vi "ZLIB Open Zip Archive__ogtk.vi"(4 "error in (no error)":errorcluster, 6 "append (create new)":T1, 7 "archive name":path) -> (0 "error out":errorcluster, 2 "globalComment":string, 3 "zip Refnum":T2)   [LabVIEW 2019]
doc: "Opens a zip session."
uses:
  <userlib>/_OpenG.lib/lvzip/lvzlib.dll
  ZLIB Zip Handle__ogtk.ctl
  ZLIB Open ZIP Mode__ogtk.ctl
panel:
  # "Please visit http://www.OpenG.org to learn about the\nOpen Source LabVIEW software movement.\n\nNOTICE -- YOU MUST LEAVE THIS NOTICE IN PLACE.  PER THE TERMS OF THE LICENSE BELOW, YOU MAY SUBLICENSE THIS SOFTWARE \nIN ANY WAY THAT DOES NOT CONFLICT WITH THIS LICENSE.\n\n### BSD License (http://www.opensource.org/licenses/bsd-license.php) Begin ###\n \nCopyright (C) 2002-2004 Rolf Kalbermatter rolf.kalbermatter@citeng.com\nCopyright (C) 2002 Jim Kring jim@jimkring.com\n\nAll rights reserved.\n\nRedistribution and use in source and binary forms, with or without modification, are permitted provided that the following conditions are met:\n\n    * Redistributions of source code must retain the above copyright notice, this list of conditions and the following disclaimer.\n    * Redistributions in binary form must reproduce the above copyright notice, this list of conditions and the following disclaimer in the \n       documentation and/or other materials provided with the distribution.\n    * Neither the name of SciWare, James Kring, Inc., nor the names of its contributors may be used to endorse or promote products derived \n       from this software without specific prior written permission.\n\nTHIS SOFTWARE IS PROVIDED BY THE COPYRIGHT HOLDERS AND CONTRIBUTORS \"AS IS\" AND ANY EXPRESS OR IMPLIED WARRANTIES, \nINCLUDING, BUT NOT LIMITED TO, THE IMPLIED WARRANTIES OF MERCHANTABILITY AND FITNESS FOR A PARTICULAR PURPOSE ARE \nDISCLAIMED. IN NO EVENT SHALL THE COPYRIGHT OWNER OR CONTRIBUTORS BE LIABLE FOR ANY DIRECT, INDIRECT, INCIDENTAL,\n SPECIAL, EXEMPLARY, OR CONSEQUENTIAL DAMAGES (INCLUDING, BUT NOT LIMITED TO, PROCUREMENT OF SUBSTITUTE GOODS OR \nSERVICES; LOSS OF USE, DATA, OR PROFITS; OR BUSINESS INTERRUPTION) HOWEVER CAUSED AND ON ANY THEORY OF LIABILITY, \nWHETHER IN CONTRACT, STRICT LIABILITY, OR TORT (INCLUDING NEGLIGENCE OR OTHERWISE) ARISING IN ANY WAY OUT OF THE USE \nOF THIS SOFTWARE, EVEN IF ADVISED OF THE POSSIBILITY OF SUCH DAMAGE.\n\n### BSD License End ###"
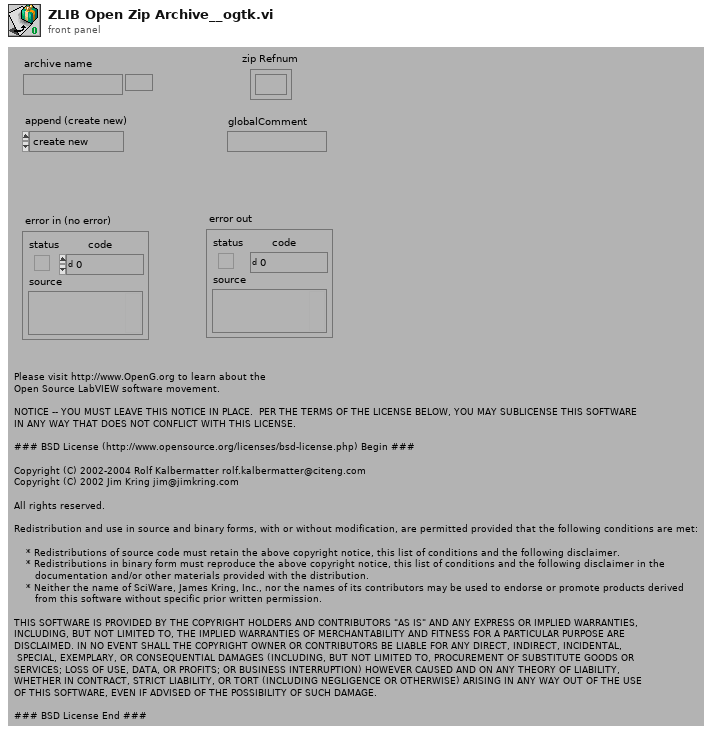
[diagram p1: front panel]
types:
  T1 = typedef "ZLIB Open ZIP Mode__ogtk.ctl" = enum16{"create new", "append to end", "append to archive"}
  T2 = typedef "ZLIB Zip Handle__ogtk.ctl" = refnum<k1>
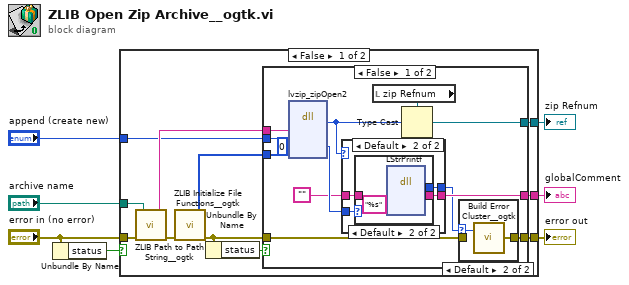
[diagram p0: block diagram]
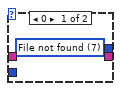
[diagram p3: hidden frame]
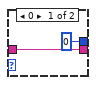
[diagram p4: hidden frame]
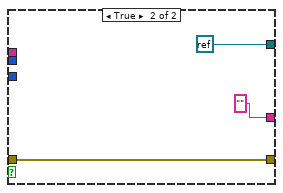
[diagram p5: hidden frame]
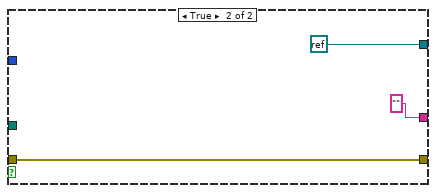
[diagram p6: hidden frame]
diagram:
  n1 = Unbundle By Name("error in (no error)") -> ("status"=w3:bool)
  n2 = case shown="False" w3 {
    tunnel: "archive name" -> [w16 _]
    tunnel: [w18 refnum<k0> refnum] -> w6
    tunnel: "error in (no error)" -> [w14 w52]
    tunnel: [w17 w52] -> w5
    tunnel: "append (create new)" -> [w13 _]
    tunnel: [w8 "" ("dest")] -> w1
    frame False {
      n3 = call "ZLIB Path to Path String__ogtk.vi"("error in (no error)"=w14, "LV file path"=w16) -> ("error in (no error)"=w11:errorcluster, "path string"=w15:string)  [unwired: 4 in]
      n4 = call "ZLIB Initialize File Functions__ogtk.vi"("error in (no error)"=w11) -> ("error out"=w10:errorcluster, "fileFuncs"=w12:u8[])  [unwired: 5 in]
      n5 = Unbundle By Name(w10) -> ("status"=w9:bool)
      n6 = case shown="False" w9 {
        tunnel: [w30 refnum<k0> refnum] -> w18
        tunnel: [w22 w49] -> w17
        tunnel: w15 -> [w28 _]
        tunnel: w13 -> [w27 _]
        tunnel: w12 -> [w26 _]
        tunnel: w10 -> [w20 w49]
        tunnel: [w23 "" ("dest")] -> w8
        frame False {
          n7 = dll-call lib="C:/Program Files (x86)/National Instruments/LabVIEW 2020/user.lib/_OpenG.lib/lvzip/lvzlib.*" fn="lvzip_zipOpen2"("path"=w28, "append"=w27, "globalComment"=u32 0, "fileFuncs"=w26) -> (w31:u32, "globalComment"=w24:u32)  [unwired: 6 in, 2 out]
          n8 = case shown="Default" w31 {
            tunnel: w24 -> [_ w39]
            tunnel: [w35 w40] -> w23
            tunnel: [w36 w38] -> w19
            tunnel: "" -> [w35 w37]
            frame 0 {
              w36 = 7 items=["No error", "Argument error", "Memory is full", "Out of zone", "End of file", "File already open", "Generic file I/O error", "File not found", "File permission error", "Disk is full", "Duplicate path", "Too many files open", "System feature not enabled", "Resource file not found", "Cannot add resource", "Resource not found", "Image not found", "Image memory error", "Pen does not exist", "Config type invalid", "Config token not found", "Config parse error", "Config memory error", "Bad external code format", "Bad external code offset", "External code not present", "Null window", "Destroy window error", "Null menu", "Print aborted", "Bad print record", "Print driver error", "Windows error during printing", "Memory error during printing", "Print dialog error", "Generic print error", "Invalid device refnum", "Device not found", "Device parameter error", "Device unit error", "Cannot open device", "Device call aborted", "Generic error", "Cancelled by user", "Object ID too low", "Object ID too high", "Object not in heap", "Unknown heap", "Unknown object (invalid DefProc)", "Unknown object (DefProc not in table)", "Message out of range", "Invalid (null) method", "Unknown message", "Manager call not supported", "Bad address", "Network operation in progress", "Network operation timed out", "Connection is busy", "Network attribute not supported", "Network error", "Address in use", "System out of memory", "Connection aborted", "Connection refused", "Not connected", "Already connected", "Connection closed", "Initialization error (interapplication manager)", "Bad occurrence", "Wait on unbound occurrence handler", "Occurrence queue overflow", "Datalog type conflict", "Unused", "Unrecognized type (interapplication manager)", "Memory corrupt", "Failed to make temporary DLL", "Old CIN version", "Drag socket not found", "Failed to load drop-object", "Failed to register OLE object", "Failed to release OLE object", "Format specifier type mismatch", "Unknown format specifier", "Too few format specifiers", "Too many format specifiers", "Scan failed", "Newer CIN version", "Error converting to variant", "Runtime menu error", "Password tampered", "Variant attribute not found", "Incompatible variant data type", "Event data is not available", "Event Store is not present", "Occurrence is not found", "Event Queue is not created", "Event info is not available", "Refnum passed is NULL", "Error retrieving Class GUID", "Error retrieving CoClass GUID", "Error retrieving TypeLib GUID.", "Bad built application magic bytes.", "Specific driver is different from the specific driver associated with the Logical Name.", "There is no session opened to the class driver.", "Max Error", "MAX - Error with config objects", "MAX - Error loading configuration", "MAX - Group not supported"]
            }
            frame Default {
              n9 = case shown="Default" w39 {
                selector: w39 -> [_ w45]
                tunnel: [w41 w47] -> w40
                tunnel: [0 w44] -> w38
                tunnel: w37 -> [w41 w43]
                frame 0 {
                }
                frame Default {
                  n10 = dll-call lib="LabVIEW" fn="LStrPrintf"("dest"=w43, "fmt"="%s", "param"=w45) -> (w44:i32, "dest"=w47:string)  [unwired: 5 in, 2 out]
                }
              }
            }
          }
          n11 = local read "zip Refnum"() -> (w29:T2)
          n12 = Type Cast(type=w29, x=w31) -> (*(type *) &x=w30:T2)
          n13 = case shown="Default" w19 {
            selector: w19 -> [_ w33]
            tunnel: [w32 w34] -> w22
            tunnel: w20 -> [w32 _]
            frame 0 {
            }
            frame Default {
              n14 = call "Build Error Cluster__ogtk.vi"("code"=w33) -> ("error out"=w34:errorcluster)  [unwired: 1 in]
            }
          }
        }
        frame True {
        }
      }
    }
    frame True {
    }
  }
  "error out" <- w5
  "zip Refnum" <- w6
  "globalComment" <- w1
